vi "exp2.vi"(0 "延时选择":i16, 1 "占空比（%）":i8, 2 "初始相位":sgl, 3 "直流偏移":sgl, 5 "停止":bool, 7 "波形选择":enum16{"正弦波", "三角波", "方波", "锯齿波"}(ring), 8 "采样频率（Hz）":sgl, 9 "频率（Hz）":dbl, 10 "幅度（V）":sgl, 11 "采样点数":i32) -> (4 "波形数据":waveform(dbl), 6 "监视器":waveform(dbl)(graph))   [LabVIEW 2022 SP3]
uses:
  <vilib>/Analysis/2dsp.llb/1D Auto Correlation (DBL).vi
  <vilib>/Analysis/NI_AALBase.lvlib
  <vilib>/Analysis/NI_AALPro.lvlib
panel:
  out "自相关":dbl[](graph)
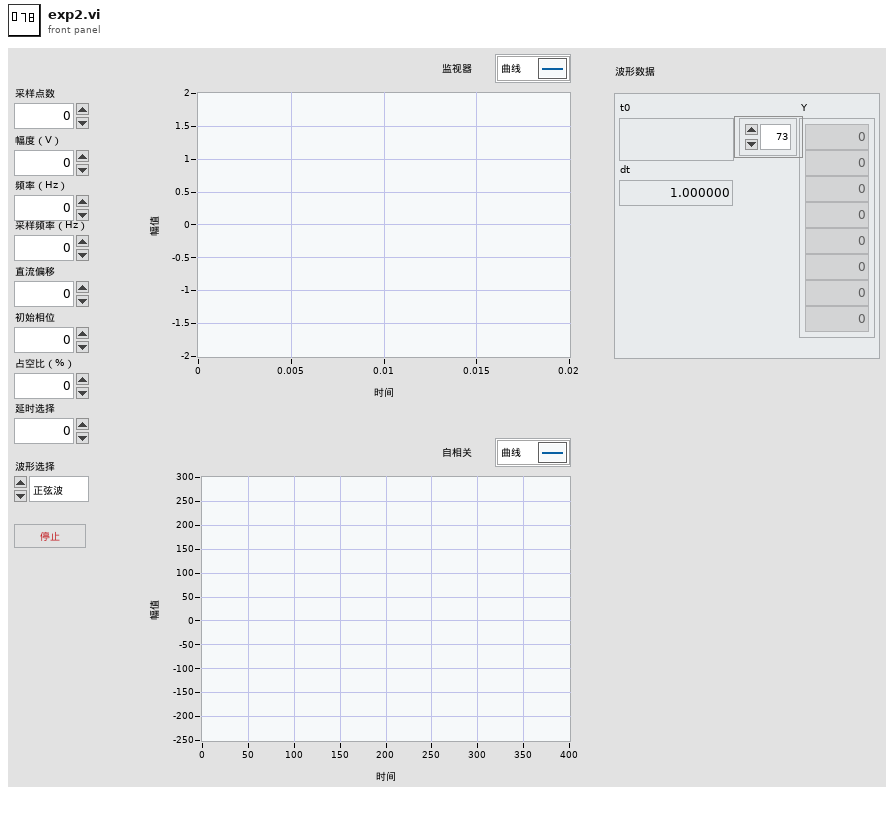
[diagram p1: front panel]
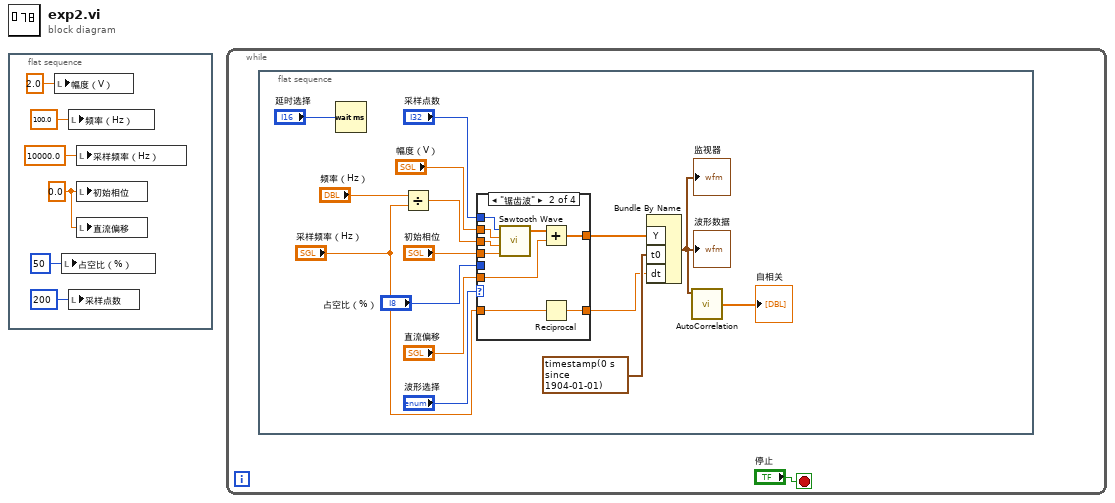
[diagram p0: block diagram]
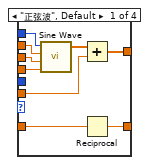
[diagram p2: hidden frame]
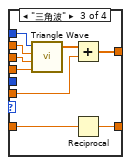
[diagram p3: hidden frame]
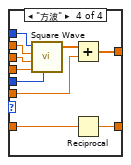
[diagram p4: hidden frame]
diagram:
  n1 = flat-sequence {
    frame #0 {
      w6 = 0.0
      n2 = local write "幅度（V）"(2.0) -> ()
      n3 = local write "占空比（%）"(50) -> ()
      n4 = local write "频率（Hz）"(100.0) -> ()
      n5 = local write "采样点数"(200) -> ()
      n6 = local write "采样频率（Hz）"(10000.0) -> ()
      n7 = local write "初始相位"(w6) -> ()
      n8 = local write "直流偏移"(w6) -> ()
    }
  }
  n9 = while {
    stop <- "停止" stop-if-true
    n10 = flat-sequence {
      frame #0 {
        n11 = Wait (ms)(milliseconds to wait="延时选择") -> ()  [unwired: 1 out]
        n12 = Divide(x="频率（Hz）", y="采样频率（Hz）") -> (x/y=w11:dbl)
        n13 = case shown="\"锯齿波\"" "波形选择" {
          tunnel: "初始相位" -> [w31 w36 w44 w55]
          tunnel: "幅度（V）" -> [w30 w32 w47 w51]
          tunnel: "采样点数" -> [w29 w33 w48 w52]
          tunnel: "采样频率（Hz）" -> [w28 w35 w45 w54]
          tunnel: "直流偏移" -> [w27 w37 w43 w56]
          tunnel: [w25 w39 w41 w57] -> w14
          tunnel: [w24 w38 w42 w58] -> w12
          tunnel: w11 -> [w23 w34 w46 w53]
          tunnel: "占空比（%）" -> [_ _ _ w50]
          frame "正弦波", Default {
            n14 = call <vilib>:"Sine Wave.vi"("samples"=w29, "amplitude"=w30, "frequency"=w23, "phase in"=w31) -> ("sine wave"=w26:dbl[])  [unwired: 1 in, 2 out]
            n15 = Add(x=w26, y=w27) -> (x+y=w25:dbl[])
            n16 = Reciprocal(x=w28) -> (1/x=w24:sgl)
          }
          frame "锯齿波" {
            n17 = call <vilib>:"Sawtooth Wave.vi"("samples"=w33, "amplitude"=w32, "frequency"=w34, "phase in"=w36) -> ("sawtooth wave"=w40:dbl[])  [unwired: 1 in, 2 out]
            n18 = Add(x=w40, y=w37) -> (x+y=w39:dbl[])
            n19 = Reciprocal(x=w35) -> (1/x=w38:sgl)
          }
          frame "三角波" {
            n20 = call <vilib>:"Triangle Wave.vi"("samples"=w48, "amplitude"=w47, "frequency"=w46, "phase in"=w44) -> ("triangle wave"=w49:dbl[])  [unwired: 1 in, 2 out]
            n21 = Add(x=w49, y=w43) -> (x+y=w41:dbl[])
            n22 = Reciprocal(x=w45) -> (1/x=w42:sgl)
          }
          frame "方波" {
            n23 = call <vilib>:"Square Wave.vi"("samples"=w52, "amplitude"=w51, "frequency"=w53, "duty cycle (%)"=w50, "phase in"=w55) -> ("square wave"=w59:dbl[])  [unwired: 1 in, 2 out]
            n24 = Add(x=w59, y=w56) -> (x+y=w57:dbl[])
            n25 = Reciprocal(x=w54) -> (1/x=w58:sgl)
          }
        }
        n26 = Bundle By Name("Y"=w14, "t0"=timestamp(0 s since 1904-01-01), "dt"=w12) -> (w8:waveform(dbl))  [unwired: 1 in]
        "监视器" <- w8
        "波形数据" <- w8
        n27 = call-poly <vilib>:"AutoCorrelation.vi"("X"=w8) -> ("Rxx"=→"自相关":dbl[])  [unwired: 9 in, 1 out]
      }
    }
  }
